vi "HQ Main.vi"() -> ()   [LabVIEW 2014]
uses:
  Type Defs/PodHealth.ctl
  Sensors/IMU - Adafruit BNO055/IMU Control.ctl
panel:
  out "Pressure":dbl(slide)=100000.0 scale=0.0..100000.0 scale format="%#_6p"
  in  "Phase":T1={"Pre-Flight Tests"=FALSE, "Accelerate"=TRUE, "Coast"=FALSE, "Brake"=FALSE, "Rest & Remove"=FALSE}
  in  "Detail Window":enum32{"Detailed Telemetry", "Configuration"}(tab)
  out "V & P Monitor":cluster{"Voltage (Total)":dbl, "Power":dbl}(graph)={"Voltage (Total)"=11.91201, "Power"=9.516504789}
  in  "Position":T2={"Maglock Max (mm)"=3.0, "Maglock Min (mm)"=0.0, "Lev. Min (mm)"=8.0, "Lev. Max (mm)"=15.0}
  in  "Pressure":T3={"HP Max (PSI)"=3000.0, "HP Min (PSI)"=2000.0, "MP Max (PSI)"=350.0, "MP Min (PSI)"=250.0, "LP Max (PSI)"=55.0, "LP Min (PSI)"=45.0}
  in  "Power 2":T4={"Brake Max (mA)"=400.0, "Brake Min (mA)"=200.0, "Batt. Min (V)"=11.5, "Batt. Max (V)"=13.0}
  in  "Stop":bool
  out "Power":dbl(knob)=9.144776890538314 scale=0.0..10.0
  out "Voltage":dbl(knob)=11.942438656676648 scale=11.0..12.0
  out "Temp1":dbl(slide)=81.63265306122449 scale=0.0..100.0
  in  "Sensor Power":bool=TRUE
  out "Laser Position":T5={"Laser 1"=FALSE, "Count 1"=23, "Laser 2"=FALSE, "Count 2"=23}
  out "IMU":T6 {"Gyroscope"."Z" scale=-45.0..45.0; "Gyroscope"."Y" scale=-45.0..45.0; "Gyroscope"."X" scale=-45.0..45.0; "Magnetometer"."Z" scale=-2500.0..2500.0; "Magnetometer"."Y" scale=-2500.0..2500.0; "Magnetometer"."X" scale=-2500.0..2500.0; "Accelerometer"."Z" scale=-5.0..5.0; "Accelerometer"."Y" scale=-5.0..5.0; "Accelerometer"."X" scale=-5.0..5.0}
  out "Gap 4":u8(slide)=11 scale=0.0..100.0
  out "Gap 3":u8(slide)=10 scale=0.0..200.0
  out "Gap 2":u8(slide)=12 scale=0.0..100.0
  out "Maglock 1":u8(slide) scale=0.0..100.0
  out "Gap 1":u8(slide)=13 scale=0.0..100.0
  in  "Track Position":dbl(slide)=438.0053908355795 scale=0.0..5000.0
  out "Pod Health":T7={"Overall Pod Health"=TRUE, "Power"={"Power"=TRUE, "Friction Brakes"=TRUE, "Magnetic Brakes"=TRUE, "Primary Battery"=TRUE, "Backup Battery"=TRUE}, "Pressure"={"Pressure"=TRUE, "HP"=TRUE, "MP "=TRUE, "LP"=TRUE}, "Position"={"Position"=TRUE, "Maglock"=TRUE, "Levitation (ToF)"=TRUE}}
  # "Live Feed"
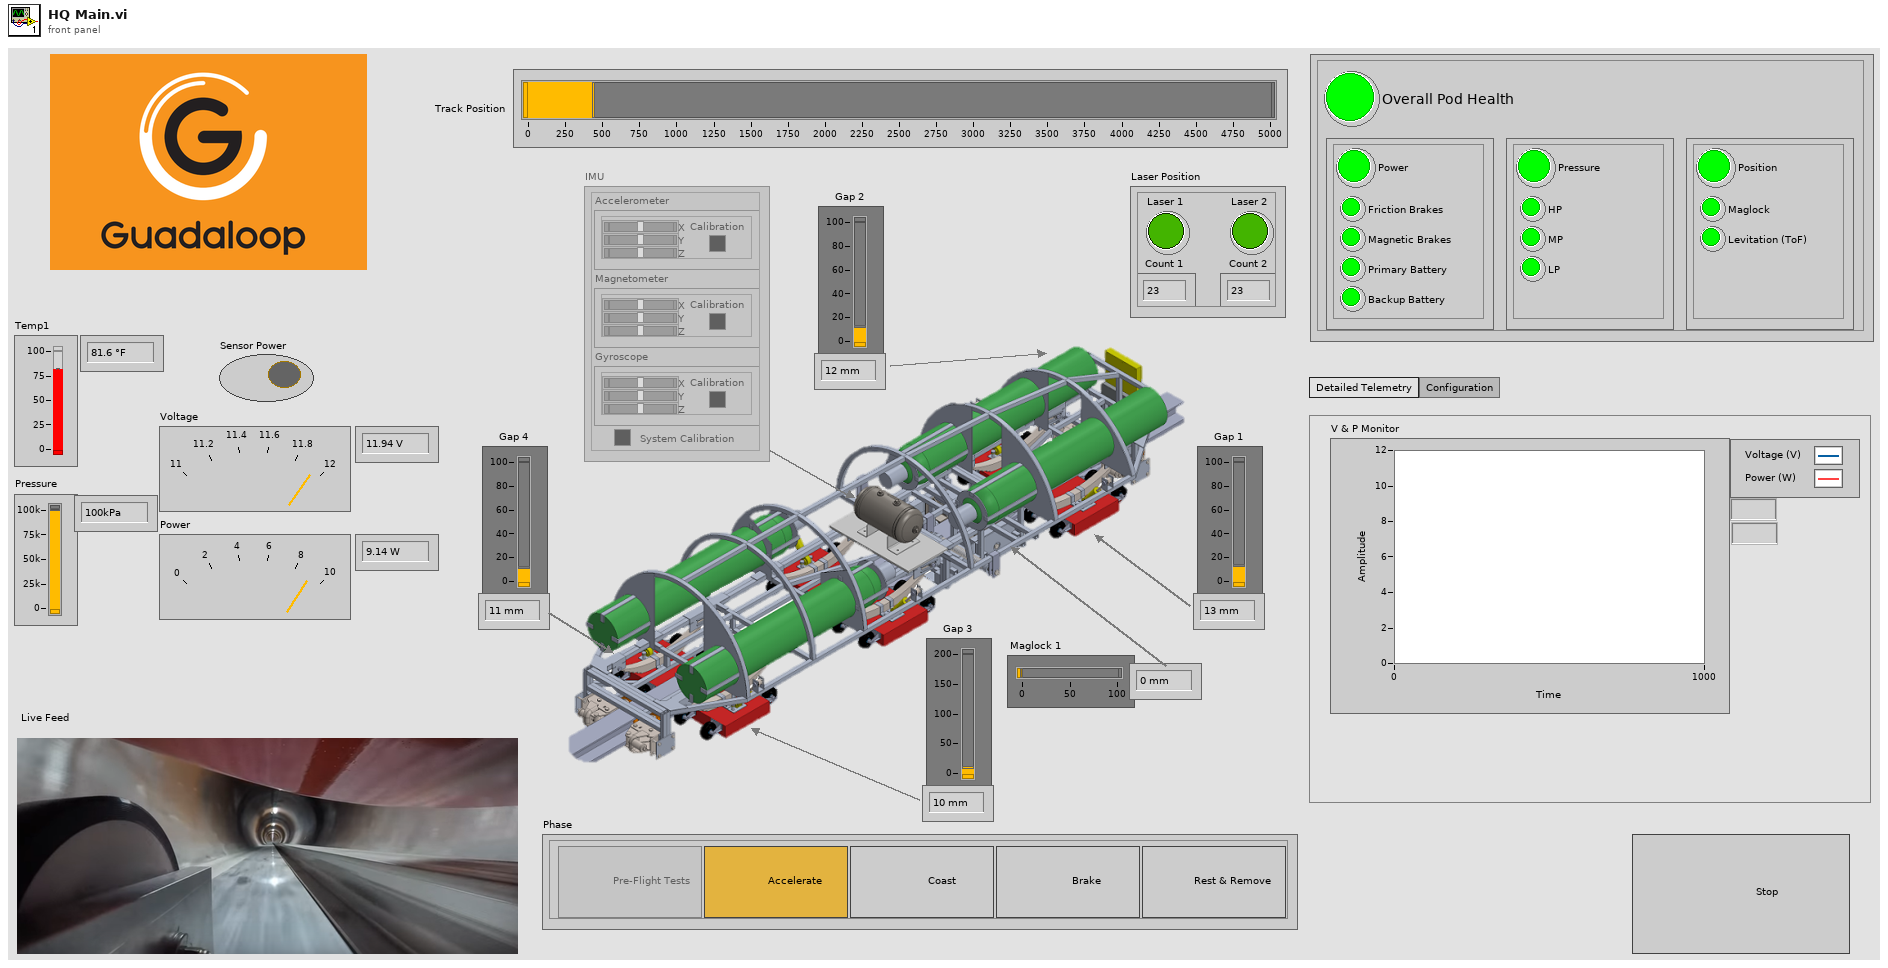
[diagram p1: front panel]
types:
  T1 = cluster{"Pre-Flight Tests":bool, "Accelerate":bool, "Coast":bool, "Brake":bool, "Rest & Remove":bool}
  T2 = cluster{"Maglock Max (mm)":dbl, "Maglock Min (mm)":dbl, "Lev. Min (mm)":dbl, "Lev. Max (mm)":dbl}
  T3 = cluster{"HP Max (PSI)":dbl, "HP Min (PSI)":dbl, "MP Max (PSI)":dbl, "MP Min (PSI)":dbl, "LP Max (PSI)":dbl, "LP Min (PSI)":dbl}
  T4 = cluster{"Brake Max (mA)":dbl, "Brake Min (mA)":dbl, "Batt. Min (V)":dbl, "Batt. Max (V)":dbl}
  T5 = cluster{"Laser 1":bool, "Count 1":u32, "Laser 2":bool, "Count 2":u32}
  T6 = typedef "IMU Control.ctl" = cluster{"Accelerometer":cluster{"X":dbl, "Y":dbl, "Z":dbl, "Calibration":u32}, "Magnetometer":cluster{"X":dbl, "Y":dbl, "Z":dbl, "Calibration":u32}, "Gyroscope":cluster{"X":dbl, "Y":dbl, "Z":dbl, "Calibration":u32}, "System Calibration":u32}
  T7 = typedef "PodHealth.ctl" = cluster{"Overall Pod Health":bool, "Power":cluster{"Power":bool, "Friction Brakes":bool, "Magnetic Brakes":bool, "Primary Battery":bool, "Backup Battery":bool}, "Pressure":cluster{"Pressure":bool, "HP":bool, "MP ":bool, "LP":bool}, "Position":cluster{"Position":bool, "Maglock":bool, "Levitation (ToF)":bool}}
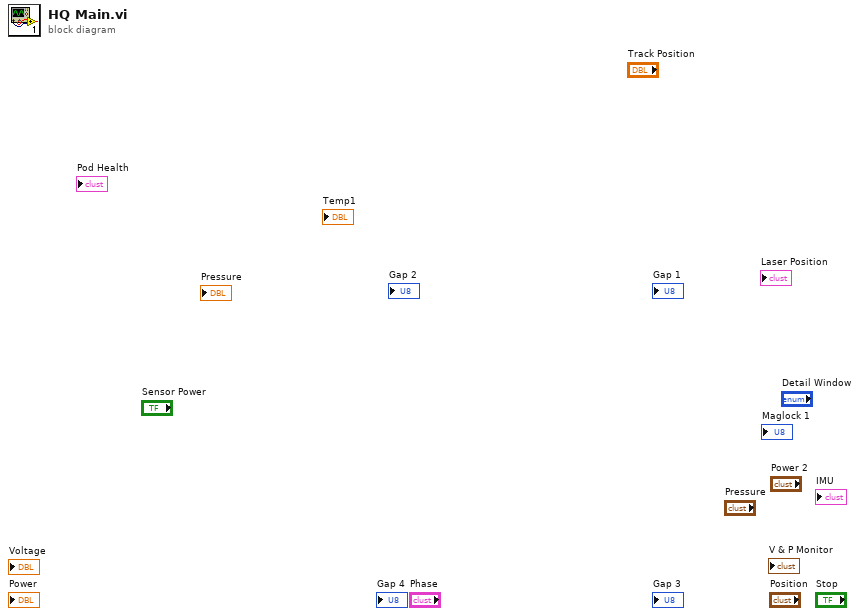
[diagram p0: block diagram]
diagram:
